vi "Graph and List Display UI.vi"() -> ()   [LabVIEW 2016]
uses:
  X-DAQ Viewer/SubVIs/Select Point Mode.ctl
  Ctrls/Select Point Operations.ctl
  Ctrls/Continuous Operations.ctl
  X-DAQ Viewer/Controls/ConfigFGVCtrl.ctl
  HardWare/Ctrls/HardWare Globals.vi
  Ctrls/GlobeVaribles.vi
  Architecture/Queue Management/ARC_Queue Destroy_Single.vi
  X-DAQ Viewer/PanelSplit/PanelSplitForDisplay.lvclass
  X-DAQ Viewer/SubVIs/New_GraphDispWithTime.vi
  X-DAQ Viewer/PanelSplit/PanelDataNode/PanelDataNode.lvclass
panel:
  in  "StartAuto":bool
  in  "StopAuto":bool
  in  "PauseAuto":bool
  in  "Stop Mannual":bool
  in  "Load":bool
  in  "save":bool
  in  "Exit":bool
  in  "ChangeUI":bool
  in  "Stop":bool
  in  "Run":bool
  in  "Pause":bool
  in  "StopManual":bool
  in  "SelectMode":enum32{"Manual", "Auto"}(radio)=enum."Auto"
  in  "Parameter":cluster{"Q-Local":string, "Variant":variant}
  in  "AdujstSplit":bool
  in  "Clear":bool
  in  "DeletePage":bool
  in  "Page":u16(ring) items=["Page0"]
  in  "AddPage":bool
  in  "ProductID":string caption="产品ID："
  in  "ManualSelect":bool
  in  "DeletePanel":bool
  in  "AddPanel":bool
  in  "Chlist":string(tree)
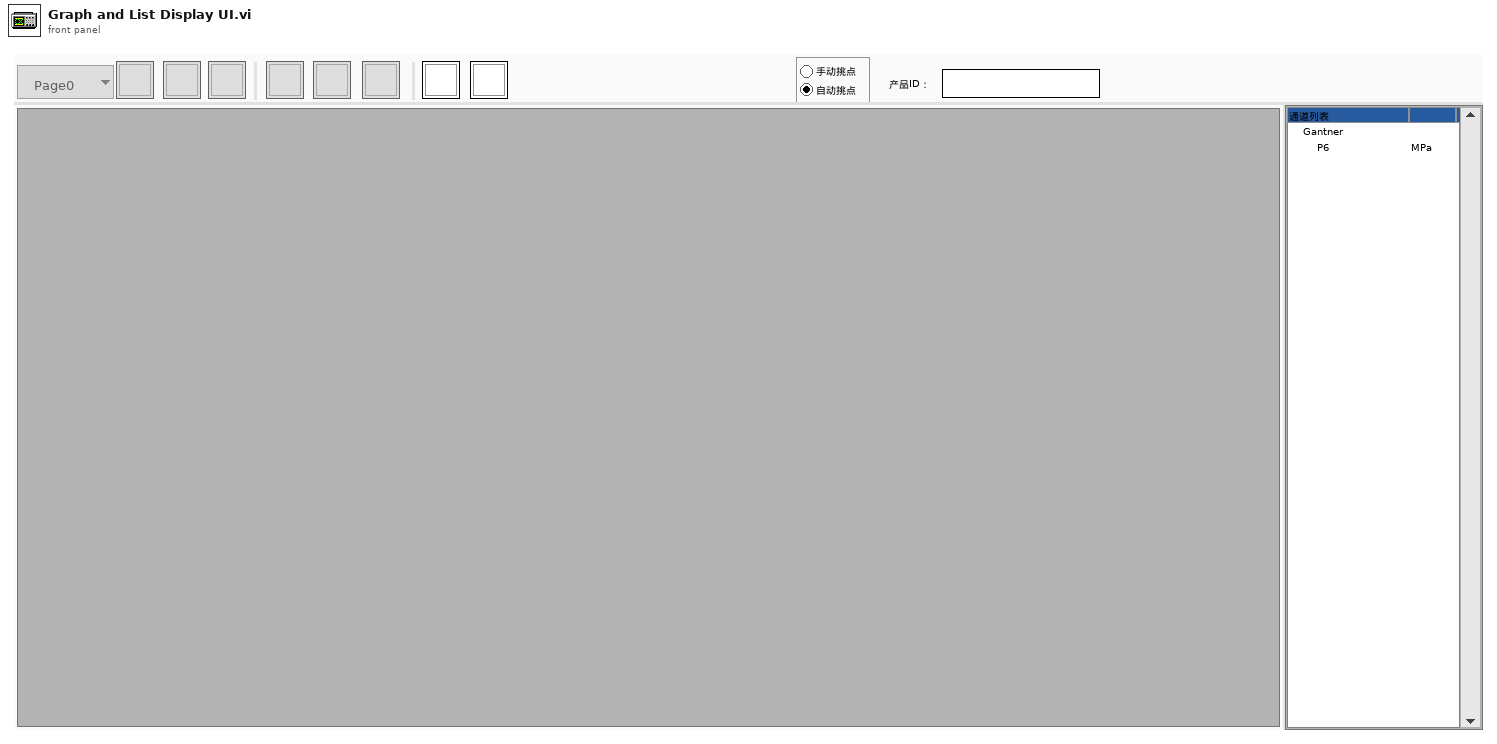
[diagram p1: front panel]
types:
  T1 = typedef "PSVCH_All Channels.ctl" = cluster{"Card Name":string, "Channels Tag":string[], "Channels Name":string[], "Type":variant[], "Uplimits":dbl[]}
  T2 = cluster{"error":errorcluster, "Q_Local Event":string, "Q_Local Data":variant, "Q_Local":string, "DAQ Channels":T1[], "Status":string, "VCHList":T1, "Q_Caller":string, "Q_PageEngine":string, "Refs":cluster{"ListUIRef":refnum<vi>, "GraphPanel":refnum<vi>, "CurrentValueUI":refnum<vi>, "PageEngineRef":refnum<vi>}, "PanelButtonsRefs":refnum<vi>[], "LoadData":string[], "UsedChList[]":cluster{"ModuTag":string, "ModuAlias":string, "ChanTag[]":string[], "ChanAlias[]":string[], "ChanUnit[]":string[]}[]}
  T3 = typedef "Select Point Operations.ctl" = enum16{"ChangeMode", "StartAuto", "PauseAuto", "StopAuto"}
  T4 = enum8{"Enabled", "Disabled", "Disabled and Grayed Out"}
  T5 = typedef "LVPoint32TypeDef.ctl" = cluster{"Horizontal":i32, "Vertical":i32}
  T6 = cluster{"data name":string, "drag data":variant}[]
  T7 = typedef "Select Point Mode.ctl" = i32
  T8 = typedef "Global para Config.ctl" = cluster{"Timing":cluster{"SampleRate":i32}, "SavePara":cluster{"FlowDiskMode":T9, "SelectMode":T7, "FolderPath":path, "Filename":string, "FileNote":string, "AutoInterval":i32, "Template":path}, "ConfigDS Path*":path, "Tdms Ref*":refnum<k34>}
  T9 = typedef "File Save Mode.ctl" = i32
  T10 = typedef "Continuous Operations.ctl" = enum16{"Writting", "Pause", "Stop"}
  T11 = typedef "ConfigFGVCtrl.ctl" = enum16{"Initialize", "Get Value", "Set Value", "Search Info"}
  T12 = cluster{"Run":refnum<vi>, "Pause":refnum<vi>, "Stop":refnum<vi>}
  T13 = cluster{"SelectMode":refnum<vi>, "ManualSelect":refnum<vi>, "StopManual":refnum<vi>, "StopAuto":refnum<vi>, "PauseAuto":refnum<vi>, "StartAuto":refnum<vi>}
  T14 = cluster{"Page":refnum<vi>, "RootPanel":refnum<vi>}
  T15 = cluster{"ModuTag":string, "ModuAlias":string, "ChanTag[]":string[], "ChanAlias[]":string[], "ChanUnit[]":string[]}[]
  T16 = typedef "HardWare _ Channel Info.ctl" = cluster{"PhyCHtags[]":string[], "VCHTags":string[], "AllNames":string[], "AllAlias":string[], "AllUnits":string[], "AllName(Unit)":string[], "AllAlarmMax":dbl[], "AllAlarmMin":dbl[], "VCHFormula[]":string[], "VCHAlias[]":string[]}
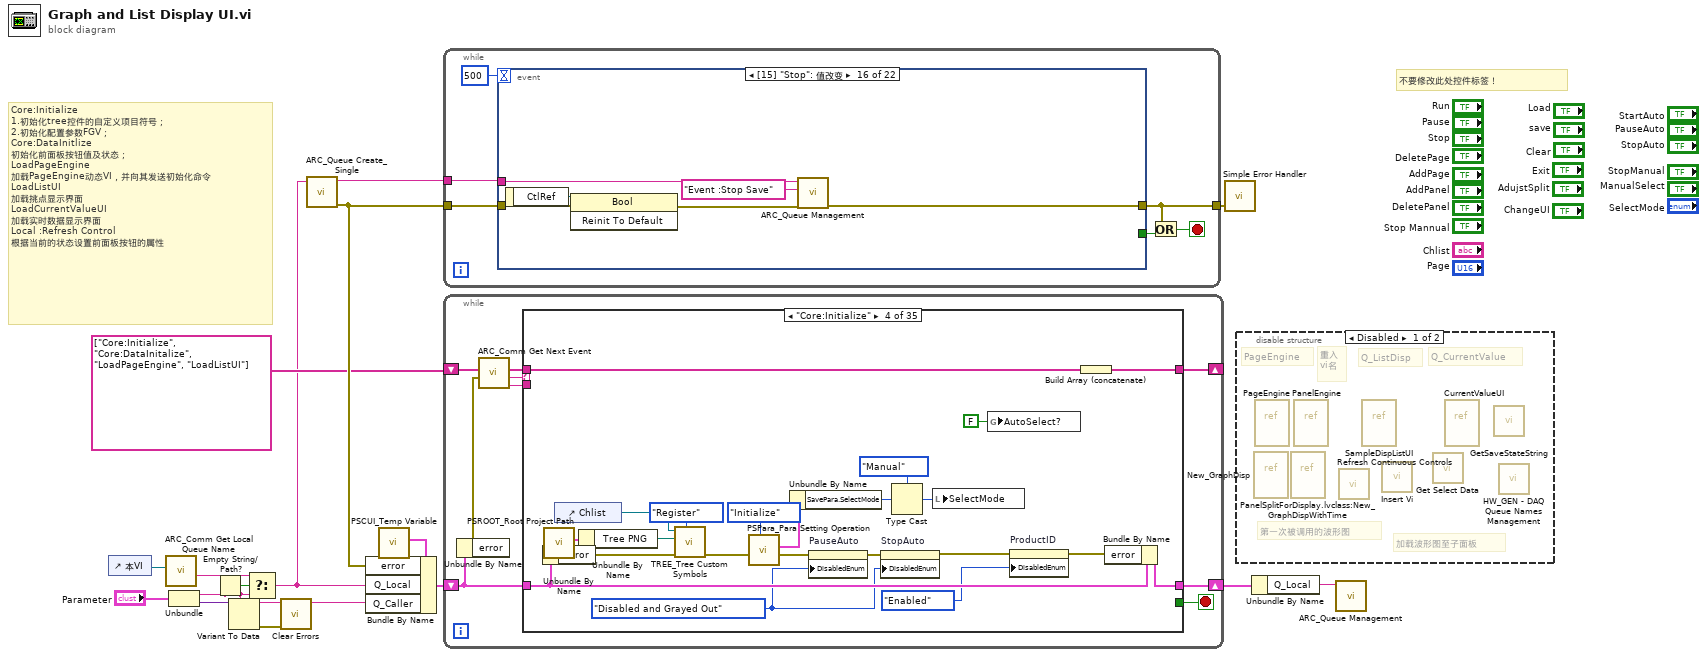
[diagram p0: block diagram]
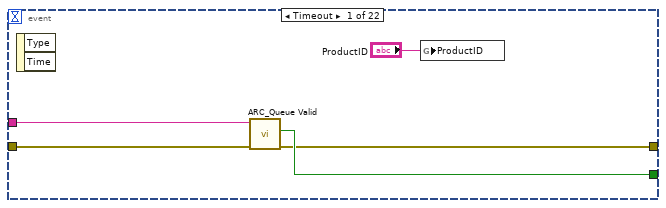
[diagram p3: hidden frame]
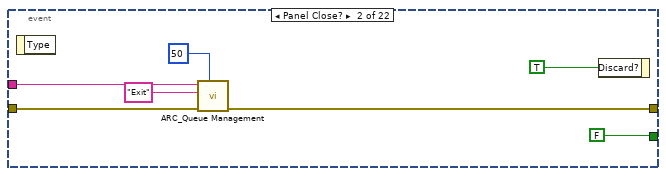
[diagram p4: hidden frame]
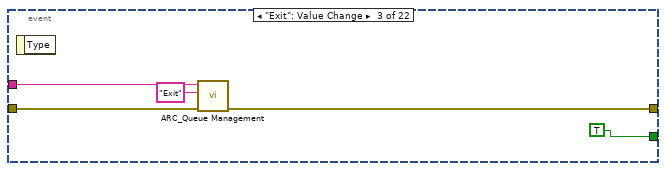
[diagram p5: hidden frame]
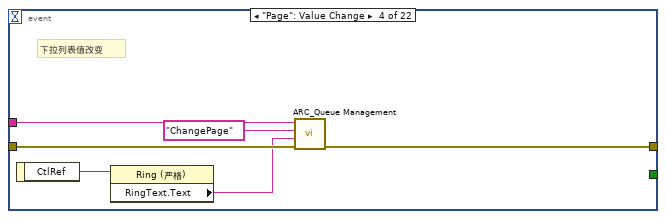
[diagram p6: hidden frame]
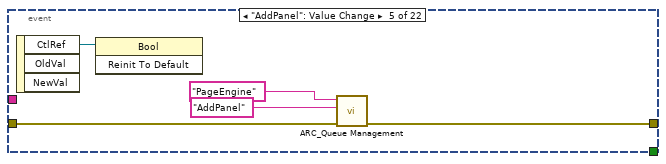
[diagram p7: hidden frame]
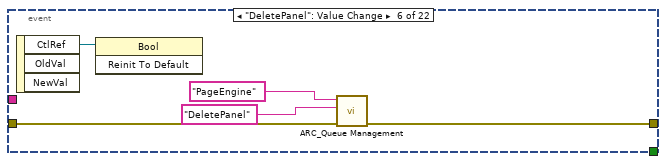
[diagram p8: hidden frame]
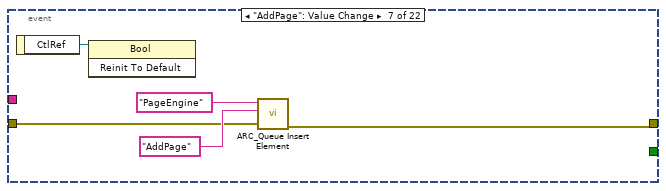
[diagram p9: hidden frame]
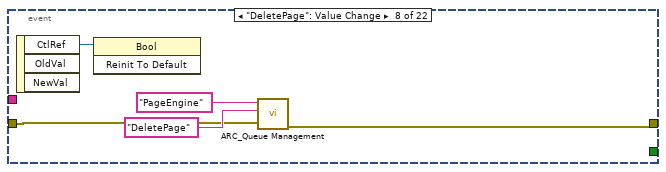
[diagram p10: hidden frame]
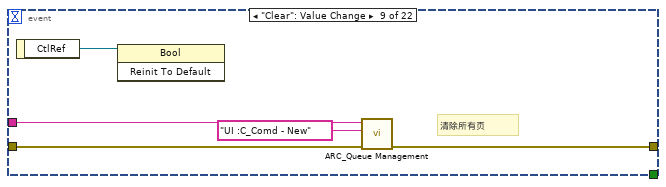
[diagram p11: hidden frame]
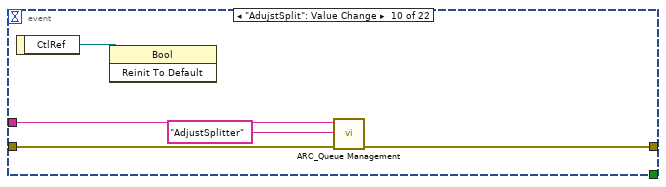
[diagram p12: hidden frame]
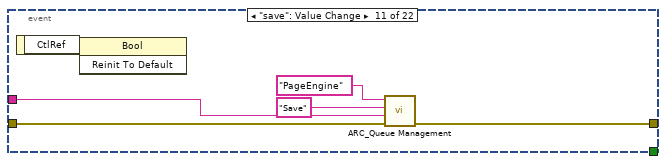
[diagram p13: hidden frame]
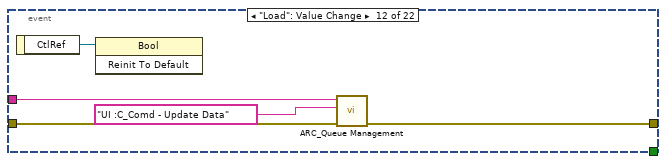
[diagram p14: hidden frame]
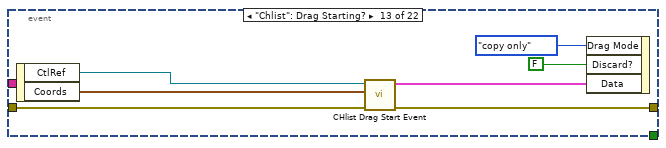
[diagram p15: hidden frame]
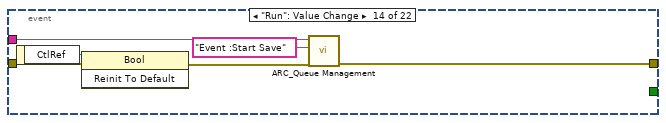
[diagram p16: hidden frame]
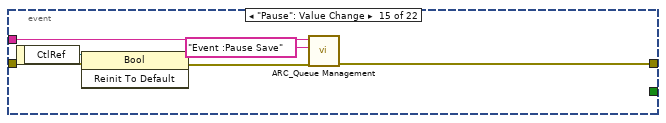
[diagram p17: hidden frame]
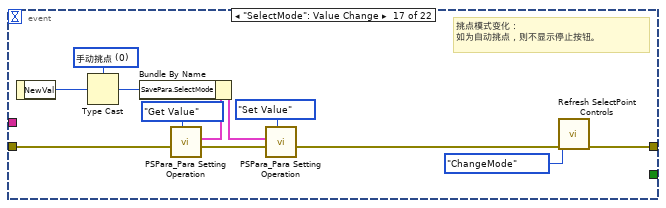
[diagram p18: hidden frame]
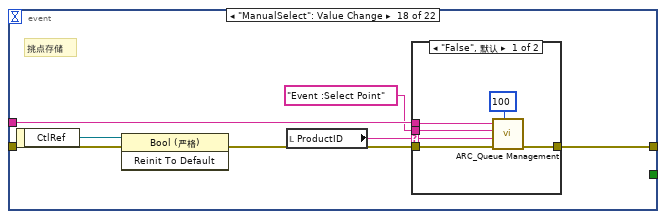
[diagram p19: hidden frame]
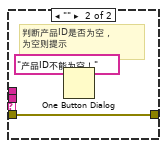
[diagram p20: hidden frame]
diagram:
  # "Core:Initialize\n1.初始化tree控件的自定义项目符号；\n2.初始化配置参数FGV；\nCore:DataInitlize\n初始化前面板按钮值及状态；\nLoadPageEngine\n加载PageEngine动态VI，并向其发送初始化命令\nLoadListUI\n加载挑点显示界面\nLoadCurrentValueUI\n加载实时数据显示界面\nLocal :Refresh Control\n根据当前的状态设置前面板按钮的属性"
  # "不要修改此处控件标签！"
  n1 = control-ref of="本VI"() -> (w9:refnum<vi>)
  n2 = call "ARC_Comm Get Local Queue Name.vi"("VI Ref"=w9) -> ("VI  Name"=w7:string)  [unwired: 8 in, 2 out]
  n3 = Unbundle("Parameter") -> ("Q-Local"=w3:string, "Variant"=w2:variant)
  n4 = Empty String/Path?(string/path=w3) -> (empty?=w8:bool)
  n5 = Variant To Data(type=w3, Variant=w2) -> (data=w5:string, error out=w4:errorcluster)  [unwired: 1 in]
  n6 = Select(t=w7, s=w8, f=w3) -> (s? t:f=w6:string)
  n7 = call <vilib>:"Clear Errors.vi"("error in (no error)"=w4) -> ()  [unwired: 5 in, 2 out]
  n8 = call "ARC_Queue Create_Single.vi"("Queue Name"=w6) -> ("error out"=w13:errorcluster, "Queue Name dup"=w11:string)  [unwired: 8 in, 1 out]
  n9 = call "PSCUI_Temp Variable.vi"() -> ("TmpData"=w12:T2)  [unwired: 11 in]
  n10 = Bundle By Name(cluster=w12, "error"=w13, "Q_Local"=w6, "Q_Caller"=w5) -> (w15:T2)
  n11 = while {
    tunnel: w13 -> [w22]
    tunnel: w11 -> [w23]
    tunnel: [w19] -> w16
    stop <- w20 stop-if-true
    n12 = event shown="[15] \"Stop\": 值改变" {
      selector: _ -> [_ _ _ _ _ _ _ _ _ _ _ _ _ _ _ _ _ _ _ _ _ _]
      dyn-events: _ -> [_ _ _ _ _ _ _ _ _ _ _ _ _ _ _ _ _ _ _ _ _ _]
      timeout: 500 -> [_ _ _ _ _ _ _ _ _ _ _ _ _ _ _ _ _ _ _ _ _ _]
      tunnel: [w26 FALSE TRUE _ _ _ _ _ _ _ _ _ _ _ _ _ _ _ _ _ _ _] -> w21
      tunnel: w23 -> [w28 w34 w39 w41 _ _ _ _ w69 w73 w77 w83 _ w99 w105 w111 _ w131 w146 w162 w168 w170]
      tunnel: w22 -> [w27 w33 w38 w46 w48 w53 w57 w64 w71 w76 w79 w85 w91 w96 w102 w108 w124 w128 w142 w159 w167 w172]
      tunnel: [w24 w32 w37 w45 w47 w52 w59 w63 w70 w75 w78 w84 w90 w100 w106 w112 w114 w127 w145 w156 w164 w171] -> w19
      event Timeout {
        n13 = event-data() -> ()  [unwired: 1 in, 2 out]
        n14 = call "ARC_Queue Valid.vi"("error in (no error)"=w27, "Queue Name(unamed)"=w28) -> ("error out"=w24:errorcluster, "Not Exist?"=w26:bool)  [unwired: 7 in, 1 out]
        n15 = global write "HardWare Globals.vi" "ProductID"("ProductID") -> ()
      }
      event Panel Close? {
        n16 = event-data() -> ()  [unwired: 1 in, 1 out]
        n17 = call-poly "ARC_Queue Management.vi"("Time out(-1)_queue in"=50, "error in (no error)"=w33, "Event"="Exit", "Queue Name(unamed)"=w34) -> ("error out"=w32:errorcluster)  [unwired: 6 in, 1 out]
        n18 = event-data("Discard?"=TRUE ("放弃？")) -> ()  [unwired: 1 in, 1 out]
      }
      event "Exit": Value Change {
        n19 = event-data() -> ()  [unwired: 1 in, 1 out]
        n20 = call-poly "ARC_Queue Management.vi"("error in (no error)"=w38, "Event"="Exit", "Queue Name(unamed)"=w39) -> ("error out"=w37:errorcluster)  [unwired: 7 in, 1 out]
      }
      event "Page": Value Change {
        # "下拉列表值改变"
        n21 = event-data() -> ("CtlRef"=w43:refnum<vi>)  [unwired: 1 in]
        n22 = property class="Ring (严格)"(reference=w43) -> ("RingText.Text"=w42:string)  [unwired: 1 in, 2 out]
        n23 = call-poly "ARC_Queue Management.vi"("error in (no error)"=w46, "Data"=w42, "Event"="ChangePage", "Queue Name(unamed)"=w41) -> ("error out"=w45:errorcluster)  [unwired: 6 in, 1 out]
      }
      event "AddPanel": Value Change {
        n24 = event-data() -> ("CtlRef"=w49:refnum<vi>)  [unwired: 1 in, 2 out]
        n25 = invoke class="Bool" method="Reinit To Default"(reference=w49) -> ()  [unwired: 2 in, 3 out]
        n26 = call-poly "ARC_Queue Management.vi"("error in (no error)"=w48, "Event"="AddPanel", "Queue Name(unamed)"="PageEngine" ("QueueName")) -> ("error out"=w47:errorcluster)  [unwired: 7 in, 1 out]
      }
      event "DeletePanel": Value Change {
        n27 = event-data() -> ("CtlRef"=w54:refnum<vi>)  [unwired: 1 in, 2 out]
        n28 = invoke class="Bool" method="Reinit To Default"(reference=w54) -> ()  [unwired: 2 in, 3 out]
        n29 = call-poly "ARC_Queue Management.vi"("error in (no error)"=w53, "Event"="DeletePanel", "Queue Name(unamed)"="PageEngine" ("QueueName")) -> ("error out"=w52:errorcluster)  [unwired: 7 in, 1 out]
      }
      event "AddPage": Value Change {
        n30 = event-data() -> ("CtlRef"=w58:refnum<vi>)  [unwired: 1 in]
        n31 = invoke class="Bool" method="Reinit To Default"(reference=w58) -> ()  [unwired: 2 in, 3 out]
        n32 = call "ARC_Queue Insert Element.vi"("error in (no error)"=w57, "Event"="AddPage", "Queue Name(unamed)"="PageEngine" ("QueueName")) -> ("error out"=w59:errorcluster)  [unwired: 7 in, 1 out]
      }
      event "DeletePage": Value Change {
        n33 = event-data() -> ("CtlRef"=w62:refnum<vi>)  [unwired: 1 in, 2 out]
        n34 = invoke class="Bool" method="Reinit To Default"(reference=w62) -> ()  [unwired: 2 in, 3 out]
        n35 = call-poly "ARC_Queue Management.vi"("error in (no error)"=w64, "Event"="DeletePage", "Queue Name(unamed)"="PageEngine" ("QueueName")) -> ("error out"=w63:errorcluster)  [unwired: 7 in, 1 out]
      }
      event "Clear": Value Change {
        # "清除所有页"
        n36 = event-data() -> ("CtlRef"=w67:refnum<vi>)  [unwired: 1 in]
        n37 = invoke class="Bool" method="Reinit To Default"(reference=w67) -> ()  [unwired: 2 in, 3 out]
        n38 = call-poly "ARC_Queue Management.vi"("error in (no error)"=w71, "Event"="UI :C_Comd - New", "Queue Name(unamed)"=w69) -> ("error out"=w70:errorcluster)  [unwired: 7 in, 1 out]
      }
      event "AdujstSplit": Value Change {
        n39 = event-data() -> ("CtlRef"=w72:refnum<vi>)  [unwired: 1 in]
        n40 = invoke class="Bool" method="Reinit To Default"(reference=w72) -> ()  [unwired: 2 in, 3 out]
        n41 = call-poly "ARC_Queue Management.vi"("error in (no error)"=w76, "Event"="AdjustSplitter", "Queue Name(unamed)"=w73) -> ("error out"=w75:errorcluster)  [unwired: 7 in, 1 out]
      }
      event "save": Value Change {
        n42 = event-data() -> ("CtlRef"=w80:refnum<vi>)  [unwired: 1 in]
        n43 = invoke class="Bool" method="Reinit To Default"(reference=w80) -> ()  [unwired: 2 in, 3 out]
        n44 = call-poly "ARC_Queue Management.vi"("error in (no error)"=w79, "Data"=w77, "Event"="Save", "Queue Name(unamed)"="PageEngine" ("QueueName")) -> ("error out"=w78:errorcluster)  [unwired: 6 in, 1 out]
      }
      event "Load": Value Change {
        n45 = event-data() -> ("CtlRef"=w86:refnum<vi>)  [unwired: 1 in]
        n46 = invoke class="Bool" method="Reinit To Default"(reference=w86) -> ()  [unwired: 2 in, 3 out]
        n47 = call-poly "ARC_Queue Management.vi"("error in (no error)"=w85, "Event"="UI :C_Comd - Update Data", "Queue Name(unamed)"=w83) -> ("error out"=w84:errorcluster)  [unwired: 7 in, 1 out]
      }
      event "Chlist": Drag Starting? {
        n48 = event-data() -> ("CtlRef"=w94:refnum<vi>, "Coords"=w92:T5)  [unwired: 1 in]
        n49 = call "CHlist Drag Start Event.vi"("error in"=w91, "Coords"=w92, "TreeControl in"=w94) -> ("error out"=w90:errorcluster, "data"=w93:T6)  [unwired: 7 in]
        n50 = event-data("Drag Mode"=enum32{"copy or move", "copy only", "move only"}."copy only", "Discard?"=FALSE, "Data"=w93) -> ()  [unwired: 1 in, 1 out]
      }
      event "Run": Value Change {
        n51 = event-data() -> ("CtlRef"=w97:refnum<vi>)  [unwired: 1 in]
        n52 = invoke class="Bool" method="Reinit To Default"(reference=w97, error in=w96) -> (error out=w95:errorcluster)  [unwired: 1 in, 2 out]
        n53 = call-poly "ARC_Queue Management.vi"("error in (no error)"=w95, "Event"="Event :Start Save", "Queue Name(unamed)"=w99) -> ("error out"=w100:errorcluster)  [unwired: 7 in, 1 out]
      }
      event "Pause": Value Change {
        n54 = event-data() -> ("CtlRef"=w103:refnum<vi>)  [unwired: 1 in]
        n55 = invoke class="Bool" method="Reinit To Default"(reference=w103, error in=w102) -> (error out=w101:errorcluster)  [unwired: 1 in, 2 out]
        n56 = call-poly "ARC_Queue Management.vi"("error in (no error)"=w101, "Event"="Event :Pause Save", "Queue Name(unamed)"=w105) -> ("error out"=w106:errorcluster)  [unwired: 7 in, 1 out]
      }
      event "Stop": Value Change {
        n57 = event-data() -> ("CtlRef"=w109:refnum<vi>)  [unwired: 1 in]
        n58 = invoke class="Bool" method="Reinit To Default"(reference=w109, error in=w108) -> (error out=w107:errorcluster)  [unwired: 1 in, 2 out]
        n59 = call-poly "ARC_Queue Management.vi"("error in (no error)"=w107, "Event"="Event :Stop Save", "Queue Name(unamed)"=w111) -> ("error out"=w112:errorcluster)  [unwired: 7 in, 1 out]
      }
      event "SelectMode": Value Change {
        w119 = T7 0 items=["手动挑点", "自动挑点"] ("SavePara.SelectPointMode")
        # "挑点模式变化：\n如为自动挑点，则不显示停止按钮。"
        n60 = event-data() -> ("NewVal"=w121:enum32{"Manual", "Auto"})  [unwired: 1 in]
        n61 = Type Cast(type=w119, x=w121) -> (*(type *) &x=w120:T7)
        n62 = call "PSPara_Para Setting Operation.vi"("Operation"=enum16{"Set Value", "Get Value", "Initialize"}."Get Value", "error in"=w124) -> ("error out"=w118:errorcluster, "_Para"=w122:T8)  [unwired: 8 in]
        n63 = Bundle By Name(cluster=w122, "SavePara.SelectMode"=w120) -> (w116:T8)
        n64 = call "PSPara_Para Setting Operation.vi"("Operation"=enum16{"Set Value", "Get Value", "Initialize"}."Set Value", "error in"=w118, "_Para"=w116) -> ("error out"=w115:errorcluster)  [unwired: 7 in, 1 out]
        n65 = call "Refresh SelectPoint Controls.vi"("error in"=w115, "Cmd"=Select_Point_Operations."ChangeMode") -> ("error out"=w114:errorcluster)  [unwired: 9 in]
      }
      event "ManualSelect": Value Change {
        # "挑点存储"
        n66 = event-data() -> ("CtlRef"=w129:refnum<vi>)  [unwired: 1 in]
        n67 = invoke class="Bool (严格)" method="Reinit To Default"(reference=w129, error in=w128) -> (error out=w130:errorcluster)  [unwired: 1 in, 2 out]
        n68 = local read "ProductID"() -> (w125:string)
        n69 = case shown="\"False\", 默认" w125 {
          selector: w125 -> [w133 _]
          tunnel: w131 -> [w137 _]
          tunnel: w130 -> [w136 w139]
          tunnel: [w134 w139] -> w127
          tunnel: "Event :Select Point" ("Event") -> [w132 _]
          frame "False", Default {
            n70 = call-poly "ARC_Queue Management.vi"("Time out(-1)_queue in"=100, "error in (no error)"=w136, "Data"=w133, "Event"=w132, "Queue Name(unamed)"=w137) -> ("error out"=w134:errorcluster)  [unwired: 5 in, 1 out]
          }
          frame "" {
            # "判断产品ID是否为空，\n为空则提示"
            n71 = One Button Dialog(message="产品ID不能为空！") -> ()  [unwired: 1 in, 1 out]
          }
        }
      }
      event "StartAuto": Value Change {
        # "开始自动挑点存储"
        n72 = event-data() -> ("CtlRef"=w141:refnum<vi>)  [unwired: 1 in]
        n73 = invoke class="Bool (严格)" method="Reinit To Default"(reference=w141, error in=w142) -> (error out=w140:errorcluster)  [unwired: 1 in, 2 out]
        n74 = local read "ProductID"() -> (w144:string)
        n75 = case shown="\"\"" w144 {
          selector: w144 -> [w148 _]
          tunnel: w146 -> [w152 _]
          tunnel: w140 -> [w151 w154]
          tunnel: [w149 w154] -> w145
          tunnel: "Event :Start Auto Select" ("Event") -> [w147 _]
          frame "False", Default {
            n76 = call-poly "ARC_Queue Management.vi"("Time out(-1)_queue in"=100, "error in (no error)"=w151, "Data"=w148, "Event"=w147, "Queue Name(unamed)"=w152) -> ("error out"=w149:errorcluster)  [unwired: 5 in, 1 out]
          }
          frame "" {
            # "判断产品ID是否为空，\n为空则提示"
            n77 = One Button Dialog(message="产品ID不能为空！") -> ()  [unwired: 1 in, 1 out]
          }
        }
      }
      event "StopAuto", "StopManual": Value Change {
        # "停止挑点存储"
        n78 = event-data() -> ("CtlRef"=w160:refnum<vi>)  [unwired: 1 in, 2 out]
        n79 = invoke class="Bool" method="Reinit To Default"(reference=w160, error in=w159) -> (error out=w161:errorcluster)  [unwired: 1 in, 2 out]
        n80 = call-poly "ARC_Queue Management.vi"("error in (no error)"=w161, "Event"="Event :Stop Select", "Queue Name(unamed)"=w162) -> ("error out"=w157:errorcluster)  [unwired: 7 in, 1 out]
        n81 = property on="ManualSelect" class="Bool (严格)"(error in=w157, "DisabledEnum"=T4."Enabled" ("Disabled")) -> (error out=w156:errorcluster)  [unwired: 1 in, 1 out]
      }
      event "PauseAuto": Value Change {
        # "暂停自动挑点存储，主要是用来更改产品ID"
        n82 = event-data() -> ()  [unwired: 1 in, 1 out]
        n83 = call-poly "ARC_Queue Management.vi"("error in (no error)"=w167, "Event"="Event :Pause Auto Select", "Queue Name(unamed)"=w168) -> ("error out"=w165:errorcluster)  [unwired: 7 in, 1 out]
        n84 = property on="ProductID" class="Str"(error in=w165, "DisabledEnum"=T4."Enabled" ("Disabled")) -> (error out=w164:errorcluster)  [unwired: 1 in, 1 out]
      }
      event "ChangeUI": Value Change {
        # "切换图形、列表显示"
        n85 = event-data() -> ("NewVal"=w169:bool)  [unwired: 1 in]
        n86 = case shown="真" w169 {
          tunnel: w172 -> [w178 w180]
          tunnel: [w177 w185] -> w171
          tunnel: w170 -> [w176 w184]
          frame False {
            n87 = property on="Page" class="Ring (严格)"() -> ("RingText.Text"=w174:string)  [unwired: 2 in, 2 out]
            n88 = call-poly "ARC_Queue Management.vi"("Time out(-1)_queue in"=100, "error in (no error)"=w178, "Data"=w174, "Event"="Event :Main-->Disp - Graph UI", "Queue Name(unamed)"=w176) -> ("error out"=w177:errorcluster)  [unwired: 5 in, 1 out]
          }
          frame True {
            n89 = vi-ref "SampleDispListUI.vi"() -> (w182:refnum<vi>)
            n90 = call "ARC_Dynamic Load by Ref.vi"("error in"=w180, "Static vi reference in"=w182) -> ("错误输出"=w179:errorcluster, "Dynamic vi reference out"=w181:refnum<vi>)  [unwired: 8 in]
            n91 = call-poly "ARC_Queue Management.vi"("error in (no error)"=w179, "Data"=w181, "Event"="Event :Main-->Disp - List UI", "Queue Name(unamed)"=w184) -> ("error out"=w185:errorcluster)  [unwired: 6 in, 1 out]
          }
        }
      }
    }
    n92 = Or(x=w19, y=w21) -> (x .or. y?=w20:bool)
  }
  n93 = while {
    shift-right: [w191] -> w17
    shift-left: w15 -> [w192]
    shift-right: [w190] -> _
    shift-left: string[] ["Core:Initialize", "Core:DataInitalize", "LoadPageEngine", "LoadListUI"] -> [w189]
    stop <- w194 stop-if-true
    n94 = Unbundle By Name(w192) -> ("error"=w193:errorcluster)
    n95 = call "ARC_Comm Get Next Event.vi"("error in (no error)"=w193, "event queue in"=w189) -> ("prev event"=w186:string, "next event"=w187:string, "event queue out"=w188:string[])  [unwired: 4 in]
    n96 = case shown="\"Core:Initialize\"" w187 {
      selector: w187 -> [w198 _ _ _ _ _ _ _ _ _ _ _ _ _ _ _ _ w388 _ _ _ _ _ _ _ _ _ _ _ _ _ _ _ _ _]
      tunnel: w188 -> [w199 w203 w227 w249 w278 w281 _ w298 w313 w321 w327 w328 w339 w358 w365 w372 w378 w392 w406 w417 w428 w429 w439 w445 w454 w456 w461 w479 w496 w508 w523 w529 w535 w545 w560]
      tunnel: w186 -> [_ _ w219 _ _ _ _ _ _ _ _ _ _ _ _ _ _ _ _ _ _ _ _ _ _ _ _ _ _ _ _ _ w530 _ _]
      tunnel: [TRUE _ _ _ _ TRUE FALSE _ _ _ _ FALSE _ _ _ _ _ _ _ _ _ _ _ _ _ _ _ _ _ _ _ _ _ _ _] -> w194
      tunnel: w192 -> [w200 w211 w226 w246 w266 w282 w292 w297 w301 w320 w326 w329 w337 w357 w370 w371 w377 w391 w405 w416 w427 w430 w438 w444 w453 w455 w464 w476 w494 w512 w519 w525 w537 w541 w556]
      tunnel: [w200 w214 w225 w247 w277 w282 w292 w297 w300 w319 w325 w329 w336 w356 w369 w371 w376 w386 w402 w414 w425 w430 w435 w443 w451 w455 w462 w475 w493 w510 w518 w524 w536 w539 w554] -> w191
      tunnel: [w199 w201 w227 w248 w278 w281 w287 w298 w313 w321 w327 w328 w339 w358 w364 w372 w378 w392 w406 w417 w428 w429 w439 w445 w454 w456 w460 w479 w496 w507 w523 w529 w535 w545 w560] -> w190
      frame Default {
        n97 = Format Into String(format string="分支\"%s\"不存在！" ("格式字符串"), w198) -> (resulting string=w197:string)  [unwired: 2 in, 1 out]
        n98 = One Button Dialog(message=w197) -> ()  [unwired: 1 in, 1 out]
      }
      frame "", "Idle" {
        n99 = Unbundle By Name(w211) -> ("Q_Caller"=w207:string, "Q_Local"=w210:string, "error"=w209:errorcluster)
        n100 = Empty String/Path?(string/path=w207) -> (empty?=w208:bool)
        n101 = case shown="假" w208 {
          tunnel: [w216 _] -> w206
          tunnel: w207 -> [w217 _]
          frame False {
            n102 = call "ARC_Queue Valid.vi"("Queue Name(unamed)"=w217) -> ("Not Exist?"=w216:bool)  [unwired: 8 in, 2 out]
          }
          frame True {
          }
        }
        n103 = call "ARC_Queue Remove Element.vi"("Time out(-1)_queue out"=100 ("Time out(-1)"), "error in (no error)"=w209, "Queue Name(unamed)"=w210) -> ("error out"=w215:errorcluster, "Data"=w213:variant, "Event"=w205:string)  [unwired: 5 in, 1 out]
        n104 = Select(t="Exit" ("Event"), s=w206, f=w205) -> (s? t:f=w202:string)
        n105 = Build Array (concatenate)(w203, w202) -> (w201:string[])
        n106 = Bundle By Name(cluster=w211, "Q_Local Data"=w213, "error"=w215) -> (w214:T2)
      }
      frame "UI:Core - Error" {
        n107 = Unbundle By Name(w226) -> ("Q_Local"=w218:string, "error"=w221:errorcluster)
        n108 = call "GEN_Error Info.vi"("error in"=w221, "Event name"=w219, "Thread name"=w218) -> ("error out"=w224:errorcluster, "Error Report"=w223:string)  [unwired: 7 in]
        n109 = call "Error Handle_Error Info insert Queue.vi"("error in"=w224, "error info in"=w223) -> ("error out"=w222:errorcluster)  [unwired: 9 in]
        n110 = call <vilib>:"Clear Errors.vi"("error in (no error)"=w222) -> ("error out"=w220:errorcluster)  [unwired: 5 in, 1 out]
        n111 = Bundle By Name(cluster=w226, "error"=w220) -> (w225:T2)
      }
      frame "Core:Initialize" {
        w232 = T4."Disabled and Grayed Out" ("Disabled")
        n112 = Unbundle By Name(w246) -> ("error"=w245:errorcluster)
        n113 = call "PSROOT_Root Project Path.vi"() -> ("All Path"=w240:cluster{"Tree PNG":path})  [unwired: 11 in]
        n114 = control-ref of="Chlist"() -> (w243:refnum<vi>)
        n115 = Unbundle By Name(w240) -> ("Tree PNG"=w242:path)
        n116 = call "TREE_Tree Custom Symbols.vi"("Operation"=enum16{"Register", "GetIndex"}."Register", "error in"=w245, "Files"=w242, "tree refnum"=w243) -> ("error out"=w239:errorcluster)  [unwired: 6 in, 1 out]
        n117 = call "PSPara_Para Setting Operation.vi"("Operation"=enum16{"Set Value", "Get Value", "Initialize"}."Initialize", "error in"=w239) -> ("error out"=w234:errorcluster, "_Para"=w238:T8)  [unwired: 8 in]
        n118 = Unbundle By Name(w238) -> ("SavePara.SelectMode"=w237:T7)
        n119 = property on="PauseAuto" class="Bool (严格)"(error in=w234, "DisabledEnum"=w232) -> (error out=w233:errorcluster)  [unwired: 1 in, 1 out]
        n120 = property on="StopAuto" class="Bool (严格)"(error in=w233, "DisabledEnum"=w232) -> (error out=w230:errorcluster)  [unwired: 1 in, 1 out]
        n121 = Type Cast(type=enum32{"Manual", "Auto"}."Manual" ("SelectMode"), x=w237) -> (*(type *) &x=w236:enum32{"Manual", "Auto"})
        n122 = local write "SelectMode"(w236) -> ()
        n123 = global write "HardWare Globals.vi" "AutoSelect?"(FALSE ("AutoSelect?")) -> ()
        n124 = property on="ProductID" class="Str"(error in=w230, "DisabledEnum"=T4."Enabled" ("Disabled")) -> (error out=w229:errorcluster)  [unwired: 1 in, 1 out]
        n125 = Build Array (concatenate)(w249) -> (w248:string[])
        n126 = Bundle By Name(cluster=w246, "error"=w229) -> (w247:T2)
      }
      frame "Core:DataInitalize" {
        w268 = FALSE ("Sample?")
        # "初始化变量"
        n127 = global write "GlobeVaribles.vi" "Sample?"(w268) -> ()
        n128 = local write "ChangeUI"(w268) -> ()
        n129 = control-ref of="Run"() -> (w264:refnum<vi>)
        n130 = control-ref of="Pause"() -> (w263:refnum<vi>)
        n131 = control-ref of="Stop"() -> (w262:refnum<vi>)
        n132 = control-ref of="SelectMode"() -> (w259:refnum<vi>)
        n133 = Bundle("Run"=w264, "Pause"=w263, "Stop"=w262) -> (w261:T12)  [unwired: 1 in]
        n134 = control-ref of="ManualSelect"() -> (w258:refnum<vi>)
        n135 = control-ref of="StopManual"() -> (w257:refnum<vi>)
        n136 = control-ref of="StopAuto"() -> (w256:refnum<vi>)
        n137 = control-ref of="PauseAuto"() -> (w255:refnum<vi>)
        n138 = control-ref of="StartAuto"() -> (w254:refnum<vi>)
        n139 = call "Refresh Continuous Controls.vi"("Cmd"=Continuous_Operations."Stop", "Ctrls"=w261) -> ()  [unwired: 9 in, 1 out]
        n140 = Bundle("SelectMode"=w259, "ManualSelect"=w258, "StopManual"=w257, "StopAuto"=w256, "PauseAuto"=w255, "StartAuto"=w254) -> (w253:T13)  [unwired: 1 in]
        n141 = control-ref of="Page"() -> (w276:refnum<vi>)
        n142 = control-ref of="AddPage"() -> (w275:refnum<vi>)
        n143 = control-ref of="DeletePage"() -> (w274:refnum<vi>)
        n144 = control-ref of="Clear"() -> (w273:refnum<vi>)
        n145 = control-ref of="AddPanel"() -> (w272:refnum<vi>)
        n146 = control-ref of="DeletePanel"() -> (w271:refnum<vi>)
        n147 = control-ref of="AdujstSplit"() -> (w270:refnum<vi>)
        n148 = call "Refresh SelectPoint Controls.vi"("Cmd"=Select_Point_Operations."ChangeMode", "Ctrls"=w253) -> ("error out"=w251:errorcluster)  [unwired: 9 in]
        n149 = call "Refresh SelectPoint Controls.vi"("error in"=w251, "Cmd"=Select_Point_Operations."StopAuto") -> ()  [unwired: 9 in, 1 out]
        n150 = Build Array(w276, w275, w274, w273, w272, w271, w270) -> (w269:refnum<vi>[])
        n151 = control-ref of="RootPanel"() -> (w265:refnum<vi>)
        n152 = for {
          tunnel: w269 -> [w280] mode=indexing
          tunnel: T4."Enabled" ("Disabled") -> [w279]
          n153 = property class="Ctl"(reference=w280, "DisabledEnum"=w279) -> ()  [unwired: 1 in, 2 out]
        }
        n154 = Bundle By Name(cluster=w266, "Refs.GraphPanel"=w265, "PanelButtonsRefs"=w269) -> (w277:T2)
      }
      frame "Core:Exit" {
      }
      frame "Exit" {
        n155 = Unbundle By Name(w292) -> ("Refs.CurrentValueUI"=w290:refnum<vi>, "Refs.GraphPanel"=w291:refnum<vi>)
        n156 = invoke class="VI" method="Abort VI"(reference=w290) -> (error out=w285:errorcluster)  [unwired: 2 in, 2 out]
        n157 = invoke class="SubPnl" method="Remove VI"(reference=w291) -> (error out=w288:errorcluster)  [unwired: 2 in, 2 out]
        n158 = Merge Errors(w285, w288) -> (w286:errorcluster)
        n159 = call <vilib>:"Clear Errors.vi"("error in (no error)"=w286) -> ("error out"=w284:errorcluster)  [unwired: 5 in, 1 out]
        n160 = call "ARC_Queue Insert Single Messenges.vi"("error in (no error)"=w284, "Order"="Exit" ("Event"), "Queue Name"="PageEngine" ("QueueName")) -> ("error out"=w289:errorcluster)  [unwired: 8 in]
        n161 = call <vilib>:"Clear Errors.vi"("error in (no error)"=w289) -> ()  [unwired: 5 in, 2 out]
        n162 = Build Array("Core:Exit" ("Remaining States")) -> (w287:string[])
      }
      frame "-------------------Load Dynamic UI------------------" {
      }
      frame "LoadPageEngine" {
        w299 = "PageEngine" ("QueueName")
        n163 = Unbundle By Name(w301) -> ("error"=w303:errorcluster)
        n164 = vi-ref "PageEngine.vi"() -> (w312:refnum<vi>)
        n165 = property class="VI"(reference=w312, error in=w303) -> (error out=w307:errorcluster, "Path"=w311:path)  [unwired: 1 out]
        n166 = call "ARC_Dynamic Load.vi"("error in"=w307, "Vi Path"=w311) -> ("错误输出"=w310:errorcluster)  [unwired: 8 in, 1 out]
        n167 = flat-sequence {
          tunnel: w310 -> [w315]
          tunnel: [w315] -> w309
          frame #0 {
            n168 = Wait (ms)(milliseconds to wait=u32 100 ("等待时间（毫秒）")) -> ()  [unwired: 1 out]
          }
        }
        n169 = control-ref of="Page"() -> (w306:refnum<vi>)
        n170 = control-ref of="RootPanel"() -> (w305:refnum<vi>)
        n171 = Bundle("Page"=w306, "RootPanel"=w305) -> (w304:T14)  [unwired: 1 in]
        n172 = call-poly "ARC_Queue Management.vi"("error in (no error)"=w309, "Data"=w304, "Event"="Initialize", "Queue Name(unamed)"=w299) -> ("error out"=w302:errorcluster)  [unwired: 6 in, 1 out]
        n173 = Bundle By Name(cluster=w301, "Q_PageEngine"=w299, "error"=w302) -> (w300:T2)
      }
      frame "LoadListUI" {
        # "装载列表显示界面UI"
        n174 = vi-ref "SampleDispListUI.vi"() -> (w318:refnum<vi>)
        n175 = call "ARC_Dynamic Load by Ref.vi"("Static vi reference in"=w318) -> ("错误输出"=w316:errorcluster, "Dynamic vi reference out"=w317:refnum<vi>)  [unwired: 9 in]
        n176 = Bundle By Name(cluster=w320, "Refs.ListUIRef"=w317, "error"=w316) -> (w319:T2)
      }
      frame "LoadCurrentValueUI" {
        # "装载列表显示界面UI"
        n177 = vi-ref "CurrentValueUI.vi"() -> (w324:refnum<vi>)
        n178 = property class="VI"(reference=w324) -> ("Path"=w323:path)  [unwired: 1 in, 2 out]
        n179 = call "ARC_Dynamic Load.vi"("Vi Path"=w323) -> ("vi reference"=w322:refnum<vi>)  [unwired: 9 in, 1 out]
        n180 = Bundle By Name(cluster=w326, "Refs.CurrentValueUI"=w322) -> (w325:T2)
      }
      frame "--------------------------User Event----------------------" {
      }
      frame "AdjustSplitter" {
        n181 = Unbundle By Name(w337) -> ("Q_PageEngine"=w334:string)
        n182 = Bundle By Name(cluster=cluster{"Event":string, "Data":variant} {"Event"="", "Data"=variant}, "Event"="AdjustSplitter") -> (w331:cluster{"Event":string, "Data":variant})
        n183 = call-poly "ARC_Queue Management.vi"("Data"=w331, "Event"="TransferToSingle", "Queue Name(unamed)"=w334) -> ("error out"=w335:errorcluster)  [unwired: 7 in, 1 out]
        n184 = Bundle By Name(cluster=w337, "error"=w335) -> (w336:T2)
      }
      frame "RefreshCHList" {
        n185 = Unbundle By Name(w357) -> ("error"=w353:errorcluster, "UsedChList[]"=w340:T15)
        n186 = control-ref of="Chlist"() -> (w343:refnum<vi>)
        n187 = call "ConfigFGV.vi"("Command"=ConfigFGVCtrl."Get Value", "error in"=w353) -> ("error out"=w345:errorcluster, "CHInfoOut"=w342:T16)  [unwired: 5 in, 3 out]
        n188 = Unbundle By Name(w342) -> ("AllName(Unit)"=w341:string[])
        n189 = property class="Tree (严格)"(reference=w343, error in=w345, "ColHdrString"=string[] ["通道列表"] ("列首字符串[]")) -> (reference out=w346:refnum<vi>, error out=w344:errorcluster)
        n190 = call "DAQ2ANA Data Interface.vi"("error in"=w344, "UsedChList[]"=w340, "Tree Ref"=w346) -> ("error out"=w352:errorcluster)  [unwired: 7 in, 1 out]
        n191 = call "SendToAllPanel.vi"("error in"=w352, "Event"="SetYScale") -> ("error out"=w348:errorcluster)  [unwired: 9 in]
        n192 = call-poly "ARC_Queue Management.vi"("error in (no error)"=w348, "Data"=w341, "Event"="Event :Disp-->ListDisp - RefreshCHList" ("QueueName"), "Queue Name(unamed)"="Q_ListDisp" ("QueueName")) -> ("error out"=w349:errorcluster)  [unwired: 6 in, 1 out]
        n193 = Bundle By Name(cluster=w357, "error"=w349) -> (w356:T2)
      }
      frame "Send Control Comd" {
        # ">> 控制指令,包括：开始，停止，暂停<<"
        n194 = Unbundle By Name(w370) -> ("Q_Local Event"=w366:string, "Q_Local Data"=w367:variant, "error"=w368:errorcluster)
        n195 = Variant To Data(error in=w368, type=w366, Variant=w367) -> (data=w361:string, error out=w362:errorcluster)
        n196 = call "PSCOMMON_Toolbar Comond.vi"("error in"=w362) -> ("error out"=w360:errorcluster)  [unwired: 10 in]
        n197 = call "SendCommand.vi"("error in (no error)"=w360, "Command"=w361) -> ("error out"=w359:errorcluster)  [unwired: 9 in]
        n198 = Bundle By Name(cluster=w370, "error"=w359, "Status"=w361) -> (w369:T2)
        n199 = Build Array (concatenate)("Local :Refresh Control" ("State(s) at Back (\"\")"), w365) -> (w364:string[])
      }
      frame "---------------------挑点存储----------------------" {
      }
      frame "Event :ManualSelect" {
        # "挑点存储：\n1、判断挑点文件是否存在，不存在则创建文件；\n2、存在则继续写入文件；"
        n200 = local read "ProductID"() -> (w374:string)
        n201 = call "SendCommand.vi"("Data"=w374, "Command"="ManualSelect") -> ("error out"=w375:errorcluster)  [unwired: 9 in]
        n202 = Bundle By Name(cluster=w377, "error"=w375) -> (w376:T2)
      }
      frame "Event :Select Point" {
        # "手动挑点"
        n203 = Unbundle By Name(w391) -> ("Q_Local Data"=w389:variant, "error"=w390:errorcluster)
        n204 = Variant To Data(error in=w390, type=w388, Variant=w389) -> (data=w381:string, error out=w383:errorcluster)
        n205 = call "Get Select Data.vi"("error in"=w383) -> ("error out"=w382:errorcluster, "data out"=w380:string[])  [unwired: 9 in]
        n206 = Bundle(w381, "data out"=w380) -> (w379:cluster{string, "data out":string[]})  [unwired: 1 in]
        n207 = call-poly "ARC_Queue Management.vi"("error in (no error)"=w382, "Data"=w379, "Event"="Event :Disp-->ListDisp - Select Point" ("QueueName"), "Queue Name(unamed)"="Q_ListDisp" ("QueueName")) -> ("error out"=w385:errorcluster)  [unwired: 6 in, 1 out]
        n208 = Bundle By Name(cluster=w391, "error"=w385) -> (w386:T2)
      }
      frame "Event :Start Auto Select" {
        # "开始自动挑点"
        n209 = Unbundle By Name(w405) -> ("Q_Local Data"=w404:variant, "error"=w401:errorcluster)
        n210 = property on="ProductID" class="Str"(error in=w401, "DisabledEnum"=T4."Disabled" ("Disabled")) -> (error out=w399:errorcluster)  [unwired: 1 in, 1 out]
        n211 = property on="PauseAuto" class="Bool (严格)"(error in=w399, "Value"=FALSE ("PauseSelect")) -> (error out=w398:errorcluster)  [unwired: 1 in, 1 out]
        n212 = call-poly "ARC_Queue Management.vi"("error in (no error)"=w398, "Data"=w404, "Event"="Event :Disp-->ListDisp - Start Auto Select" ("QueueName"), "Queue Name(unamed)"="Q_ListDisp" ("QueueName")) -> ("error out"=w395:errorcluster)  [unwired: 6 in, 1 out]
        n213 = call "Refresh SelectPoint Controls.vi"("error in"=w395, "Cmd"=Select_Point_Operations."StartAuto") -> ("error out"=w394:errorcluster)  [unwired: 9 in]
        n214 = Bundle By Name(cluster=w405, "error"=w394) -> (w402:T2)
      }
      frame "Event :Pause Auto Select" {
        # "暂停自动挑点按钮按下"
        n215 = Unbundle By Name(w416) -> ("error"=w411:errorcluster)
        n216 = call-poly "ARC_Queue Management.vi"("error in (no error)"=w411, "Event"="Event :Disp-->ListDisp - Pause Auto Select" ("QueueName"), "Queue Name(unamed)"="Q_ListDisp" ("QueueName")) -> ("error out"=w413:errorcluster)  [unwired: 7 in, 1 out]
        n217 = call "Refresh SelectPoint Controls.vi"("error in"=w413, "Cmd"=Select_Point_Operations."PauseAuto") -> ("error out"=w409:errorcluster)  [unwired: 9 in]
        n218 = property on="ProductID" class="Str"(error in=w409, "DisabledEnum"=T4."Enabled" ("Disabled")) -> (error out=w408:errorcluster)  [unwired: 1 in, 1 out]
        n219 = Bundle By Name(cluster=w416, "error"=w408) -> (w414:T2)
      }
      frame "Event :Stop Select" {
        # "停止挑点"
        n220 = Unbundle By Name(w427) -> ("error"=w424:errorcluster)  [unwired: 1 out]
        n221 = property on="ProductID" class="Str"(error in=w424, "DisabledEnum"=T4."Enabled" ("Disabled")) -> (error out=w421:errorcluster)  [unwired: 1 in, 1 out]
        n222 = call-poly "ARC_Queue Management.vi"("error in (no error)"=w421, "Event"="Event :Disp-->ListDisp - Stop Select" ("QueueName"), "Queue Name(unamed)"="Q_ListDisp" ("QueueName")) -> ("error out"=w420:errorcluster)  [unwired: 7 in, 1 out]
        n223 = call "Refresh SelectPoint Controls.vi"("error in"=w420, "Cmd"=Select_Point_Operations."StopAuto") -> ("error out"=w419:errorcluster)  [unwired: 9 in]
        n224 = Bundle By Name(cluster=w427, "error"=w419) -> (w425:T2)
      }
      frame "----------------------连续存储--------------------------" {
      }
      frame "Event :Start Save" {
        w431 = Continuous_Operations."Writting" ("Cmd")
        # "启动数据保存:\n1、创建数据文件；2、向主线程发送保存命令；"
        n225 = Unbundle By Name(w438) -> ("Q_Caller"=w432:string, "error"=w433:errorcluster)
        n226 = call "Refresh Continuous Controls.vi"("error in"=w433, "Cmd"=w431) -> ("error out"=w437:errorcluster)  [unwired: 9 in]
        n227 = global write "GlobeVaribles.vi" "Status"(w431) -> ()
        n228 = call "ARC_Queue Insert Single Messenges.vi"("error in (no error)"=w437, "Order"="Event :Disp-->M - Start Save", "Queue Name"=w432) -> ("error out"=w434:errorcluster)  [unwired: 8 in]
        n229 = Bundle By Name(cluster=w438, "error"=w434) -> (w435:T2)
      }
      frame "Event :Pause Save" {
        w441 = Continuous_Operations."Pause" ("Cmd")
        # "暂停数据保存:\n1、更新状态变量"
        n230 = Unbundle By Name(w444) -> ("error"=w442:errorcluster)
        n231 = global write "GlobeVaribles.vi" "Status"(w441) -> ()
        n232 = call "Refresh Continuous Controls.vi"("error in"=w442, "Cmd"=w441) -> ("error out"=w440:errorcluster)  [unwired: 9 in]
        n233 = Bundle By Name(cluster=w444, "error"=w440) -> (w443:T2)
      }
      frame "Event :Stop Save" {
        w447 = Continuous_Operations."Stop" ("Cmd")
        # "停止数据保存:\n1、向主线程发送停止保存命令；\n2、关闭数据文件；"
        n234 = Unbundle By Name(w453) -> ("Q_Caller"=w446:string, "error"=w449:errorcluster)
        n235 = call "Refresh Continuous Controls.vi"("error in"=w449, "Cmd"=w447) -> ("error out"=w448:errorcluster)  [unwired: 9 in]
        n236 = call "ARC_Queue Insert Single Messenges.vi"("error in (no error)"=w448, "Order"="Event :Disp-->M - Stop Save", "Queue Name"=w446) -> ("error out"=w450:errorcluster)  [unwired: 8 in]
        n237 = global write "GlobeVaribles.vi" "Status"(w447) -> ()
        n238 = Bundle By Name(cluster=w453, "error"=w450) -> (w451:T2)
      }
      frame "------------------------------Comm------------------------------" {
      }
      frame "Event :Main-->Disp - Update Channel Para" {
        n239 = Unbundle By Name(w464) -> ("UsedChList[]"=w458:T15, "Q_Local Data"=w465:variant, "error"=w466:errorcluster)
        n240 = Variant To Data(error in=w466, type=w458, Variant=w465) -> (data=w457:T15, error out=w463:errorcluster)
        n241 = Bundle By Name(cluster=w464, "UsedChList[]"=w457, "error"=w463) -> (w462:T2)
        n242 = Build Array (concatenate)("RefreshCHList" ("State(s) at Back (\"\")"), w461) -> (w460:string[])
      }
      frame "Event :Main-->Disp - Graph UI" {
        # "切换到波形图显示界面"
        n243 = Unbundle By Name(w476) -> ("PanelButtonsRefs"=w473:refnum<vi>[], "error"=w469:errorcluster)
        n244 = for {
          tunnel: w473 -> [w483] mode=indexing
          tunnel: 0 -> [w482]
          shift-right: [w481] -> w467
          shift-left: w469 -> [w480]
          n245 = property class="Ctl"(reference=w483, error in=w480, "DisabledEnum"=w482) -> (error out=w481:errorcluster)  [unwired: 1 out]
        }
        n246 = property on="Page" class="Ring (严格)"(error in=w467) -> (error out=w470:errorcluster, "RingText.Text"=w471:string)  [unwired: 1 in, 1 out]
        n247 = call-poly "ARC_Queue Management.vi"("error in (no error)"=w470, "Data"=w471, "Event"="ChangePage", "Queue Name(unamed)"="PageEngine" ("QueueName")) -> ("error out"=w474:errorcluster)  [unwired: 6 in, 1 out]
        n248 = local write "ChangeUI"(FALSE ("ChangeUI")) -> ()
        n249 = Bundle By Name(cluster=w476, "error"=w474) -> (w475:T2)
      }
      frame "Event :Main-->Disp - List UI" {
        # "切换至列表显示界面"
        n250 = Unbundle By Name(w494) -> ("PanelButtonsRefs"=w492:refnum<vi>[], "Refs.GraphPanel"=w495:refnum<vi>, "error"=w485:errorcluster)
        n251 = local write "ChangeUI"(TRUE ("ChangeUI")) -> ()
        n252 = vi-ref "SampleDispListUI.vi"() -> (w487:refnum<vi>)
        n253 = call "ARC_Dynamic Load by Ref.vi"("error in"=w485, "Static vi reference in"=w487) -> ("错误输出"=w486:errorcluster, "Dynamic vi reference out"=w484:refnum<vi>)  [unwired: 8 in]
        n254 = disable-structure shown="Enabled" {
          disable-tunnel: w495 -> [w500 _]
          disable-tunnel: [w499 w501] -> w489
          disable-tunnel: w486 -> [w498 w501]
          disable-tunnel: w484 -> [w497 _]
          frame Enabled {
            n255 = invoke class="SubPnl" method="Insert VI"(reference=w500, error in=w498, "VI Ref"=w497) -> (error out=w499:errorcluster)  [unwired: 1 in, 3 out]
          }
          frame Disabled {
          }
        }
        n256 = for {
          tunnel: w492 -> [w505] mode=indexing
          tunnel: 2 -> [w502]
          shift-right: [w504] -> w490
          shift-left: w489 -> [w503]
          n257 = property class="Ctl"(reference=w505, error in=w503, "DisabledEnum"=w502) -> (error out=w504:errorcluster)  [unwired: 1 out]
        }
        n258 = Bundle By Name(cluster=w494, "error"=w490) -> (w493:T2)
      }
      frame "ANA :C_Comd - All Channels" {
        n259 = Unbundle By Name(w512) -> ("VCHList"=w513:T1, "Q_Local Data"=w514:variant, "error"=w515:errorcluster)
        n260 = Variant To Data(error in=w515, type=w513, Variant=w514) -> (data=w509:T1, error out=w511:errorcluster)
        n261 = Bundle By Name(cluster=w512, "VCHList"=w509, "error"=w511) -> (w510:T2)
        n262 = Build Array (concatenate)("RefreshCHList" ("State(s) at Back (\"\")"), w508) -> (w507:string[])
      }
      frame "UI :C_Comd - Update Data" {
        # ">> Notes: 此处分支转发给Engine；用于文件打开。包含配置信息，一维字符串数组。<<"
        n263 = Unbundle By Name(w519) -> ("Q_PageEngine"=w522:string, "LoadData"=w517:string[], "error"=w516:errorcluster)
        n264 = call-poly "ARC_Queue Management.vi"("error in (no error)"=w516, "Data"=w517, "Event"="Load", "Queue Name(unamed)"=w522) -> ("error out"=w520:errorcluster)  [unwired: 6 in, 1 out]
        n265 = Bundle By Name(cluster=w519, "error"=w520) -> (w518:T2)
      }
      frame "UI :C_Comd - New" {
        # "清除所有页"
        # ">> Notes: 此处分支转发给Engine；用于回复初始状态。<<"
        n266 = Unbundle By Name(w525) -> ("Q_PageEngine"=w528:string)
        n267 = call-poly "ARC_Queue Management.vi"("Event"="New", "Queue Name(unamed)"=w528) -> ("error out"=w526:errorcluster)  [unwired: 8 in, 1 out]
        n268 = Bundle By Name(cluster=w525, "error"=w526) -> (w524:T2)
      }
      frame "SendToPageEngine" {
        n269 = Unbundle By Name(w537) -> ("Q_PageEngine"=w531:string, "Q_Local Data"=w533:variant, "error"=w534:errorcluster)
        n270 = call-poly "ARC_Queue Management.vi"("error in (no error)"=w534, "Data"=w533, "Event"=w530, "Queue Name(unamed)"=w531) -> ("error out"=w532:errorcluster)  [unwired: 6 in, 1 out]
        n271 = Bundle By Name(cluster=w537, "error"=w532) -> (w536:T2)
      }
      frame "Save" {
        # ">> Notes: 用于测试接收Page引擎发送过来的保存信息<<"
        n272 = Unbundle By Name(w541) -> ("Q_Local Data"=w544:variant, "error"=w542:errorcluster)
        n273 = Variant To Data(error in=w542, type=string[] [], Variant=w544) -> (data=w538:string[], error out=w540:errorcluster)
        n274 = Bundle By Name(cluster=w541, "LoadData"=w538, "error"=w540) -> (w539:T2)
      }
      frame "Write Data When Pause" {
        # ">> Notes: 此处延时存在风险；组名称是否合并？<<"
        n275 = Unbundle By Name(w556) -> ("DAQ Channels"=w550:T1[], "VCHList"=w549:T1, "error"=w558:errorcluster)
        n276 = Wait (ms)(milliseconds to wait=u32 900) -> ()  [unwired: 1 out]
        n277 = Build Array(w549) -> (w548:T1[])
        n278 = Build Array(w550, w548) -> (w547:T1[][])
        n279 = call "PSPara_Para Setting Operation.vi"("Operation"=enum16{"Set Value", "Get Value", "Initialize"}."Get Value") -> ("_Para"=w559:T8)  [unwired: 9 in, 1 out]
        n280 = Unbundle By Name(w559) -> ("Tdms Ref*"=w552:refnum<k34>, "Timing"=w557:cluster{"SampleRate":i32})
        n281 = for {
          tunnel: w557 -> [w570]
          tunnel: w552 -> [w565]
          shift-right: [w566] -> w555
          shift-left: w558 -> [w571]
          tunnel: string[] ["连续存储数据", "虚拟通道"] -> [w563] mode=indexing
          tunnel: w547 -> [w561] mode=indexing
          n282 = for {
            tunnel: [w581] -> w562 mode=concatenating
            tunnel: [w580] -> w569 mode=concatenating
            tunnel: w561 -> [w579] mode=indexing
            n283 = Unbundle By Name(w579) -> ("Channels Name"=w581:string[], "Type"=w580:variant[])
          }
          n284 = call "PSCUI_Get NaN Waveforms.vi"("error in (no error)"=w571, "Units"=w569, "Channels Name"=w562, "Timing"=w570) -> ("error out"=w568:errorcluster, "Waveforms"=w567:waveform(dbl)[])  [unwired: 6 in]
          n285 = Not A Number/Path/Refnum?(number/path/refnum=w565) -> (NaN/Path/Refnum?=w564:bool)
          n286 = case shown="假" w564 {
            tunnel: w568 -> [w577 w578]
            tunnel: w567 -> [w576 _]
            tunnel: [w575 w578] -> w566
            tunnel: w565 -> [w574 _]
            tunnel: w563 -> [w573 _]
            tunnel: w562 -> [w572 _]
            frame False {
              n287 = TDMS Write(0:w574, 5:w573, 7:w572, 9:w576, 11:w577) -> (15:w575:errorcluster)  [unwired: 1 in, 3 out]
            }
            frame True {
            }
          }
        }
        n288 = Bundle By Name(cluster=w556, "error"=w555) -> (w554:T2)
      }
    }
  }
  n289 = call <vilib>:"Simple Error Handler.vi"("error in (no error)"=w16) -> ()  [unwired: 4 in, 5 out]
  n290 = disable-structure shown="Disabled" {
    frame Disabled {
      # "加载波形图至子面板"
      # "第一次被调用的波形图"
      # "Q_CurrentValue"
      # "重入\nvi名"
      # "PageEngine"
      # "Q_ListDisp"
      n291 = vi-ref "New_GraphDisp.vi"() -> ()  [unwired: 1 out]
      n292 = vi-ref "PageEngine.vi"() -> ()  [unwired: 1 out]
      n293 = vi-ref "PanelSplitForDisplay.lvclass:New_GraphDispWithTime.vi"() -> ()  [unwired: 1 out]
      n294 = vi-ref "PanelEngine.vi"() -> ()  [unwired: 1 out]
      n295 = call "Refresh Continuous Controls.vi"() -> ()  [unwired: 11 in, 1 out]
      n296 = vi-ref "SampleDispListUI.vi"() -> ()  [unwired: 1 out]
      n297 = call-dynamic "Insert Vi.vi"() -> ()  [unwired: 10 in, 2 out]
      n298 = call "Get Select Data.vi"() -> ()  [unwired: 10 in, 2 out]
      n299 = vi-ref "CurrentValueUI.vi"() -> ()  [unwired: 1 out]
      n300 = call "GetSaveStateString.vi"() -> ()  [unwired: 10 in, 2 out]
      n301 = call "HW_GEN - DAQ Queue Names Management.vi"() -> ()  [unwired: 10 in, 2 out]
    }
    frame Enabled {
    }
  }
  n302 = Unbundle By Name(w17) -> ("Q_Local"=w14:string)
  n303 = call-poly "ARC_Queue Management.vi"("Queue Name(unamed)"=w14) -> ()  [unwired: 8 in, 3 out]
